vi "SSE.vi"(7 "LabVIEW Web Service Request":refnum<class "Web Request.lvclass">=refnum) -> ()   [LabVIEW 2015]
uses:
  <vilib>/wsapi/Web Request.lvclass
panel:
  in  "getFromVi":string="data: {\ndata: \"variable1\": \"someText\",\ndata: \"variable2\": 12345\ndata: }\n\n"
  # "Use the Web Service Request input terminal to call the VIs on the Web Services palette. Do not remove it from the connector pane unless you don't need access to the palette."
  # "Each additional control wired to the connector pane will be available as an input in the URL. To include an indicator in terminal-mode output (the default setting), it must also be wired to the connector pane."
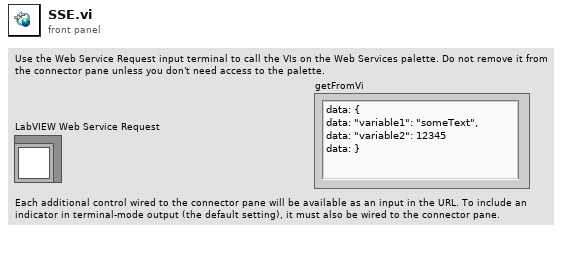
[diagram p1: front panel]
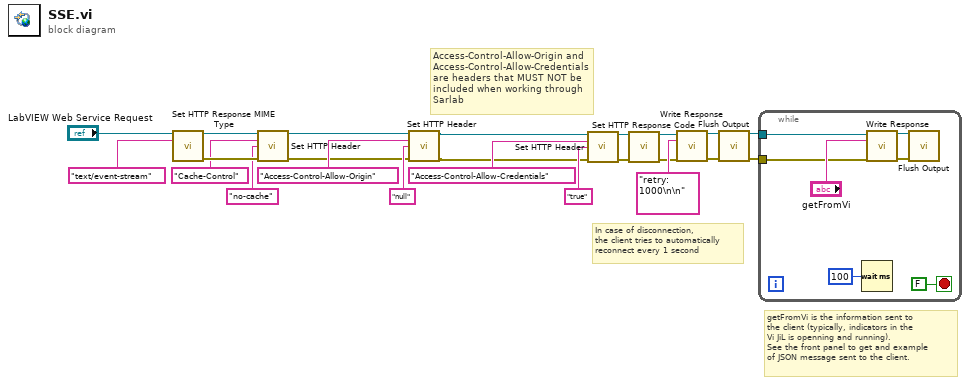
[diagram p0: block diagram]
diagram:
  # "In case of disconnection,\nthe client tries to automatically\nreconnect every 1 second"
  # "getFromVi is the information sent to\nthe client (typically, indicators in the\nVi JiL is openning and running).\nSee the front panel to get and example\nof JSON message sent to the client."
  # "Access-Control-Allow-Origin and\nAccess-Control-Allow-Credentials\nare headers that MUST NOT be\nincluded when working through\nSarlab"
  n1 = call <vilib>:"Set HTTP Response MIME Type.vi"("LabVIEW Web Service Request"="LabVIEW Web Service Request", "MIME type (text/html)"="text/event-stream" ("header")) -> ("LabVIEW Web Service Request out"=w23:refnum<class "Web Request.lvclass">, "error out"=w22:errorcluster)  [unwired: 12 in]
  n2 = call <vilib>:"Set HTTP Header.vi"("LabVIEW Web Service Request"=w23, "header"="Cache-Control", "header value"="no-cache", "error in (no error)"=w22) -> ("LabVIEW Web Service Request out"=w16:refnum<class "Web Request.lvclass">, "error out"=w15:errorcluster)  [unwired: 10 in]
  n3 = call <vilib>:"Set HTTP Header.vi"("LabVIEW Web Service Request"=w16, "header"="Access-Control-Allow-Origin", "header value"="null", "error in (no error)"=w15) -> ("LabVIEW Web Service Request out"=w8:refnum<class "Web Request.lvclass">, "error out"=w12:errorcluster)  [unwired: 10 in]
  n4 = call <vilib>:"Set HTTP Header.vi"("LabVIEW Web Service Request"=w8, "header"="Access-Control-Allow-Credentials", "header value"="true", "error in (no error)"=w12) -> ("LabVIEW Web Service Request out"=w11:refnum<class "Web Request.lvclass">, "error out"=w10:errorcluster)  [unwired: 10 in]
  n5 = call <vilib>:"Set HTTP Response Code.vi"("LabVIEW Web Service Request"=w11, "error in (no error)"=w10) -> ("LabVIEW Web Service Request out"=w4:refnum<class "Web Request.lvclass">, "error out"=w3:errorcluster)  [unwired: 12 in]
  n6 = call <vilib>:"Write Response.vi"("LabVIEW Web Service Request"=w4, "response string"="retry: 1000\n\n", "error in (no error)"=w3) -> ("LabVIEW Web Service Request out"=w6:refnum<class "Web Request.lvclass">, "error out"=w7:errorcluster)  [unwired: 11 in]
  n7 = call <vilib>:"Flush Output.vi"("LabVIEW Web Service Request"=w6, "error in (no error)"=w7) -> ("LabVIEW Web Service Request out"=w2:refnum<class "Web Request.lvclass">, "error out"=w1:errorcluster)  [unwired: 12 in]
  n8 = while {
    tunnel: w2 -> [w27]
    tunnel: w1 -> [w26]
    stop <- FALSE stop-if-true
    n9 = Wait (ms)(milliseconds to wait=u32 100) -> ()  [unwired: 1 out]
    n10 = call <vilib>:"Write Response.vi"("LabVIEW Web Service Request"=w27, "response string"="getFromVi", "error in (no error)"=w26) -> ("LabVIEW Web Service Request out"=w29:refnum<class "Web Request.lvclass">, "error out"=w30:errorcluster)  [unwired: 11 in]
    n11 = call <vilib>:"Flush Output.vi"("LabVIEW Web Service Request"=w29, "error in (no error)"=w30) -> ()  [unwired: 12 in, 2 out]
  }
